vi "PopulateParameterHyperCube.vi"(8 "error in (no error)":errorcluster, 11 "Parameter Ranges":T2[](array[typedef])) -> (0 "error out":errorcluster, 2 "2D Array":dbl[][](array[numeric]), 3 "Parameter Sequence":cluster{dbl[]}[](array[cluster]))   [LabVIEW 2019]
uses:
  ParameterRange--Cluster.ctl
panel:
  out "Range and Resolution Preview":T1(array[cluster])
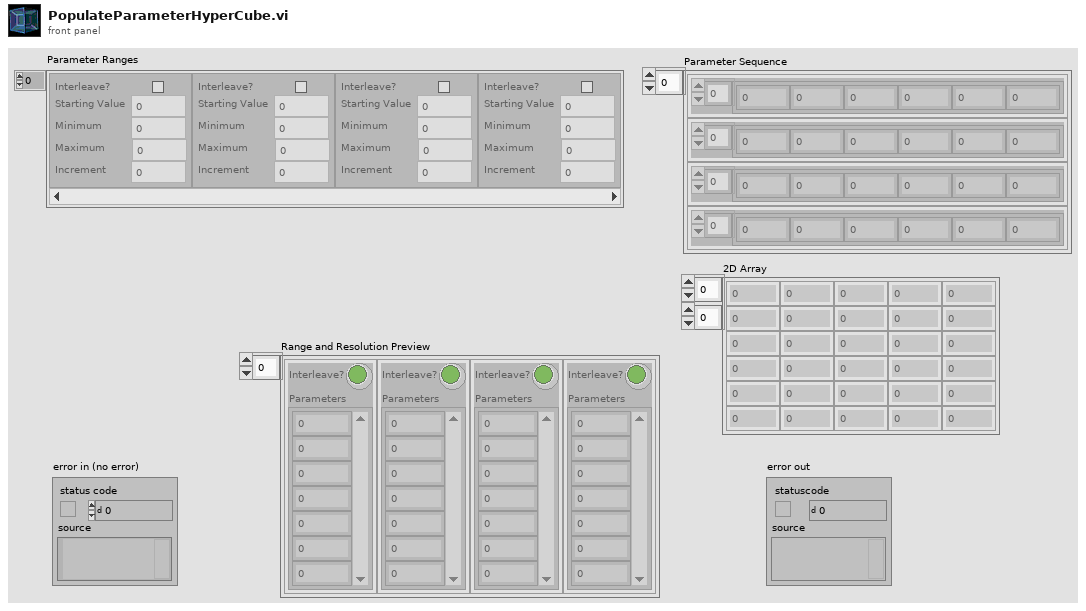
[diagram p1: front panel]
types:
  T1 = cluster{"Parameters":dbl[], "Interleave?":bool}[]
  T2 = typedef "ParameterRange--Cluster.ctl" = cluster{"Interleave?":bool, "Starting Value":dbl, "Minimum":dbl, "Maximum":dbl, "Increment":dbl}
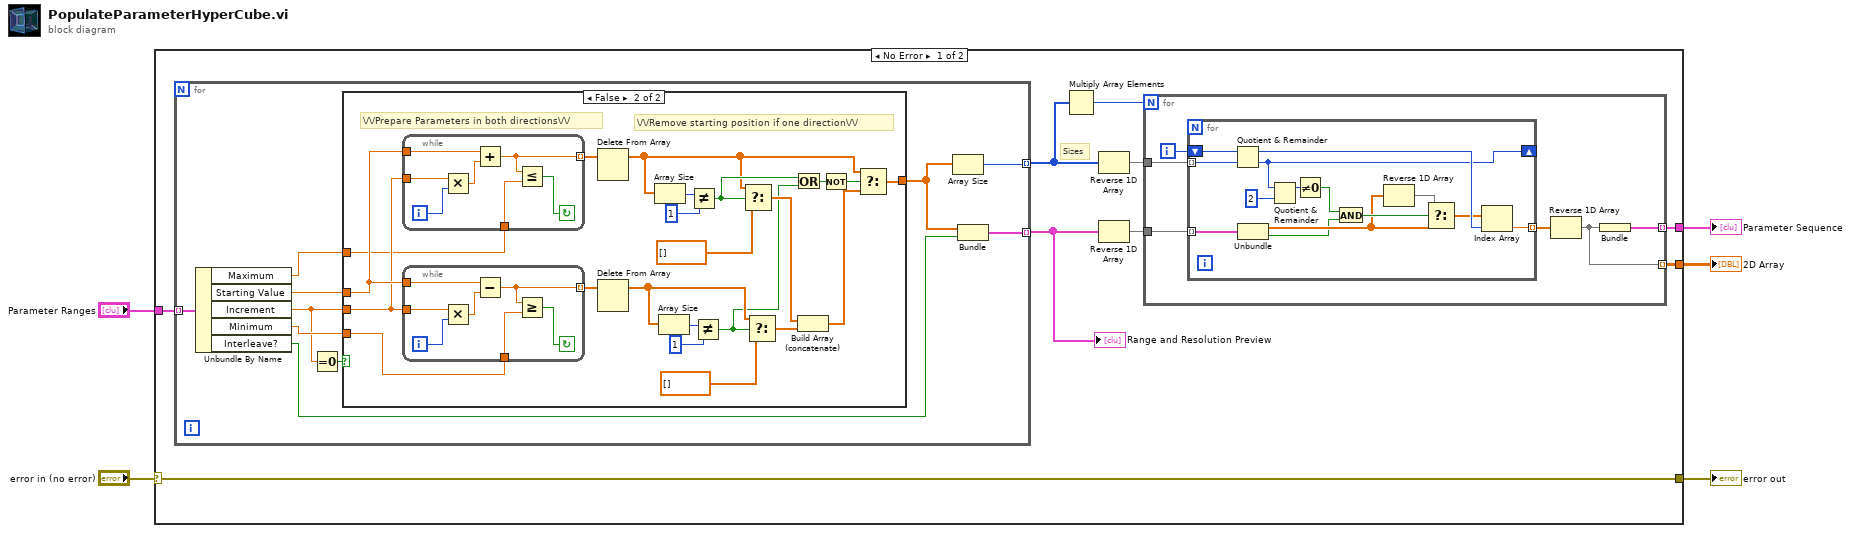
[diagram p0: block diagram]
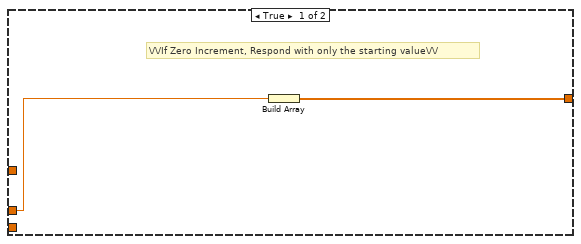
[diagram p2: hidden frame]
diagram:
  n1 = case shown="No Error" "error in (no error)" {
    selector: "error in (no error)" -> [w7 w83]
    tunnel: "Parameter Ranges" -> [w14 _]
    tunnel: [w12 _] -> w4
    tunnel: [w7 w83] -> w2
    tunnel: [w6 _] -> w1
    frame No Error {
      # "Sizes"
      n2 = for {
        tunnel: w14 -> [w24] mode=indexing
        tunnel: [w22] -> w11 mode=indexing
        tunnel: [w21] -> w10 mode=indexing
        n3 = Unbundle By Name(w24) -> ("Maximum"=w19:dbl, "Starting Value"=w23:dbl, "Increment"=w18:dbl, "Minimum"=w20:dbl, "Interleave?"=w15:bool)
        n4 = Equal To 0?(x=w18) -> (x = 0?=w17:bool)
        n5 = case shown="False" w17 {
          tunnel: w23 -> [w26 w48]
          tunnel: w18 -> [_ w45]
          tunnel: w20 -> [_ w35]
          tunnel: w19 -> [_ w34]
          tunnel: [w25 w32] -> w16
          frame True {
            # "\\/\\/If Zero Increment, Respond with only the starting value\\/\\/"
            n6 = Build Array(w26) -> (w25:dbl[])
          }
          frame False {
            # "\\/\\/Prepare Parameters in both directions\\/\\/"
            # "\\/\\/Remove starting position if one direction\\/\\/"
            n7 = while {
              tunnel: w45 -> [w62]
              tunnel: w48 -> [w60]
              tunnel: w34 -> [w58]
              tunnel: [w56] -> w46 mode=indexing
              i -> [w61]
              stop <- w57 continue-if-true
              n8 = Multiply(x=w62, y=w61) -> (x*y=w59:dbl)
              n9 = Add(x=w60, y=w59) -> (x+y=w56:dbl)
              n10 = Less Or Equal?(x=w56, y=w58) -> (x <= y?=w57:bool)
            }
            n11 = while {
              tunnel: w45 -> [w55]
              tunnel: w48 -> [w53]
              tunnel: w35 -> [w51]
              tunnel: [w49] -> w47 mode=indexing
              i -> [w54]
              stop <- w50 continue-if-true
              n12 = Multiply(x=w55, y=w54) -> (x*y=w52:dbl)
              n13 = Subtract(x=w53, y=w52) -> (x-y=w49:dbl)
              n14 = Greater Or Equal?(x=w49, y=w51) -> (x >= y?=w50:bool)
            }
            n15 = Delete From Array(array=w46) -> (array with subset deleted=w28:dbl[])  [unwired: 2 in, 1 out]
            n16 = Delete From Array(array=w47) -> (array with subset deleted=w42:dbl[])  [unwired: 2 in, 1 out]
            n17 = Array Size(array=w28) -> (size(s)=w37:i32)
            n18 = Array Size(array=w42) -> (size(s)=w44:i32)
            n19 = Not Equal?(x=w37, y=1) -> (x != y?=w31:bool)
            n20 = Not Equal?(x=w44, y=1) -> (x != y?=w30:bool)
            n21 = Select(t=w28, s=w31, f=dbl[] []) -> (s? t:f=w36:dbl[])
            n22 = Select(t=w42, s=w30, f=dbl[] []) -> (s? t:f=w41:dbl[])
            n23 = Or(x=w31, y=w30) -> (x .or. y?=w29:bool)
            n24 = Build Array (concatenate)(w36, w41) -> (w33:dbl[])
            n25 = Not(x=w29) -> (.not. x?=w27:bool)
            n26 = Select(t=w28, s=w27, f=w33) -> (s? t:f=w32:dbl[])
          }
        }
        n27 = Array Size(array=w16) -> (size(s)=w21:i32)
        n28 = Bundle(w16, "Interleave?"=w15) -> (w22:cluster{dbl[], "Interleave?":bool})  [unwired: 1 in]
      }
      "Range and Resolution Preview" <- w11
      n29 = Multiply Array Elements(1:w10) -> (0:w13:i32)
      n30 = Reverse 1D Array(array=w10) -> (reversed array=w9:i32[])
      n31 = Reverse 1D Array(array=w11) -> (reversed array=w8:cluster{dbl[], "Interleave?":bool}[])
      n32 = for {
        N: w13 -> [_]
        tunnel: w8 -> [w64]
        tunnel: w9 -> [w65]
        tunnel: [w66] -> w12 mode=indexing
        tunnel: [w63] -> w6 mode=indexing
        i -> [w68]
        n33 = for {
          tunnel: w65 -> [w82] mode=indexing
          shift-right: [w77] -> _
          shift-left: w68 -> [w81]
          tunnel: w64 -> [w80] mode=indexing
          tunnel: [w78] -> w67 mode=indexing
          n34 = Quotient & Remainder(x=w81, y=w82) -> (x-y*floor(x/y)=w79:i32, floor(x/y)=w77:i32)
          n35 = Unbundle(w80) -> (w70:dbl[], "Interleave?"=w69:bool)
          n36 = Quotient & Remainder(x=w77, y=2) -> (x-y*floor(x/y)=w75:i32)  [unwired: 1 out]
          n37 = Not Equal To 0?(x=w75) -> (x != 0?=w74:bool)
          n38 = And(x=w74, y=w69) -> (x .and. y?=w73:bool)
          n39 = Reverse 1D Array(array=w70) -> (reversed array=w72:dbl[])
          n40 = Select(t=w72, s=w73, f=w70) -> (s? t:f=w71:dbl[])
          n41 = Index Array(array=w71, index=w79) -> (element=w78:dbl)
        }
        n42 = Reverse 1D Array(array=w67) -> (reversed array=w63:dbl[])
        n43 = Bundle(w63) -> (w66:cluster{dbl[]})  [unwired: 1 in]
      }
    }
    frame Error {
    }
  }
  "Parameter Sequence" <- w4
  "error out" <- w2
  "2D Array" <- w1
